vi "test.vi"(8 "Voie physique DAQmx 2":tag="sHIT/ai0") -> ()   [LabVIEW 2013]
uses:
  <vilib>/DAQmx/read.llb/DAQmx Read (Analog Wfm 1Chan NSamp).vi
  <vilib>/DAQmx/miscellaneous.llb/DAQmx Fill In Error Info.vi
  <vilib>/express/express analysis/Spectral/Block/exnSpectralBlock spectral measurements PSD poly.vi
  <vilib>/express/express analysis/Spectral/Block/exnSpectralBlock spectral measurements PSD WFM.vi
  <vilib>/express/express analysis/Spectral/XNode/ExpressSpectralMeasurementsBlockNode.xnode
panel:
  out "Final Waveform":waveform(dbl)(graph)
  in  "Fenetre d'affichage (s)":dbl step=0.001
  out "?":cluster{"f0":dbl, "df":dbl, "magnitude":dbl[]}(graph)
  in  "FFT":bool
  out "Frequence":dbl
  out "Valeur eff":dbl
  out "Moyenne":dbl
  in  "Statistiques":bool
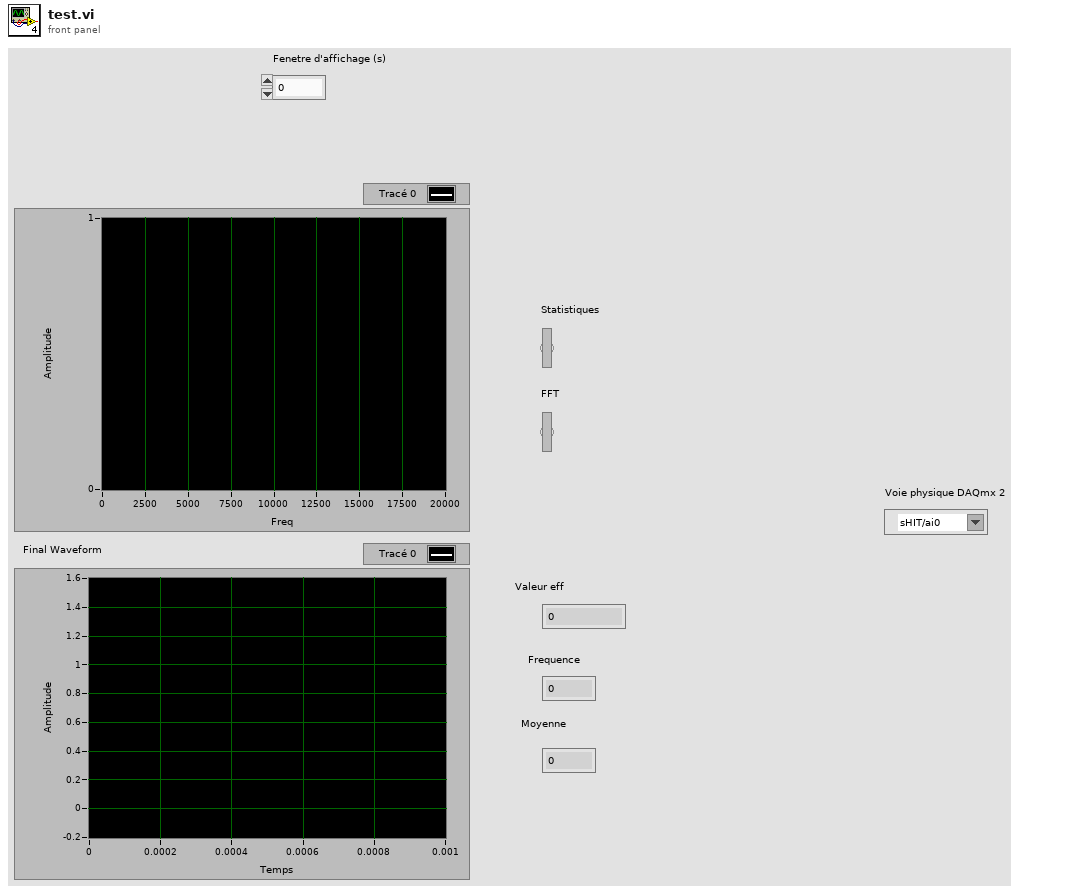
[diagram p1: front panel]
types:
  T1 = cluster{"averaging mode":u16, "weighting mode":u16, "number of averages":u32}
  T2 = cluster{"dB On (F)":bool, "unwrap phase (F)":bool, "convert to degree (F)":bool}
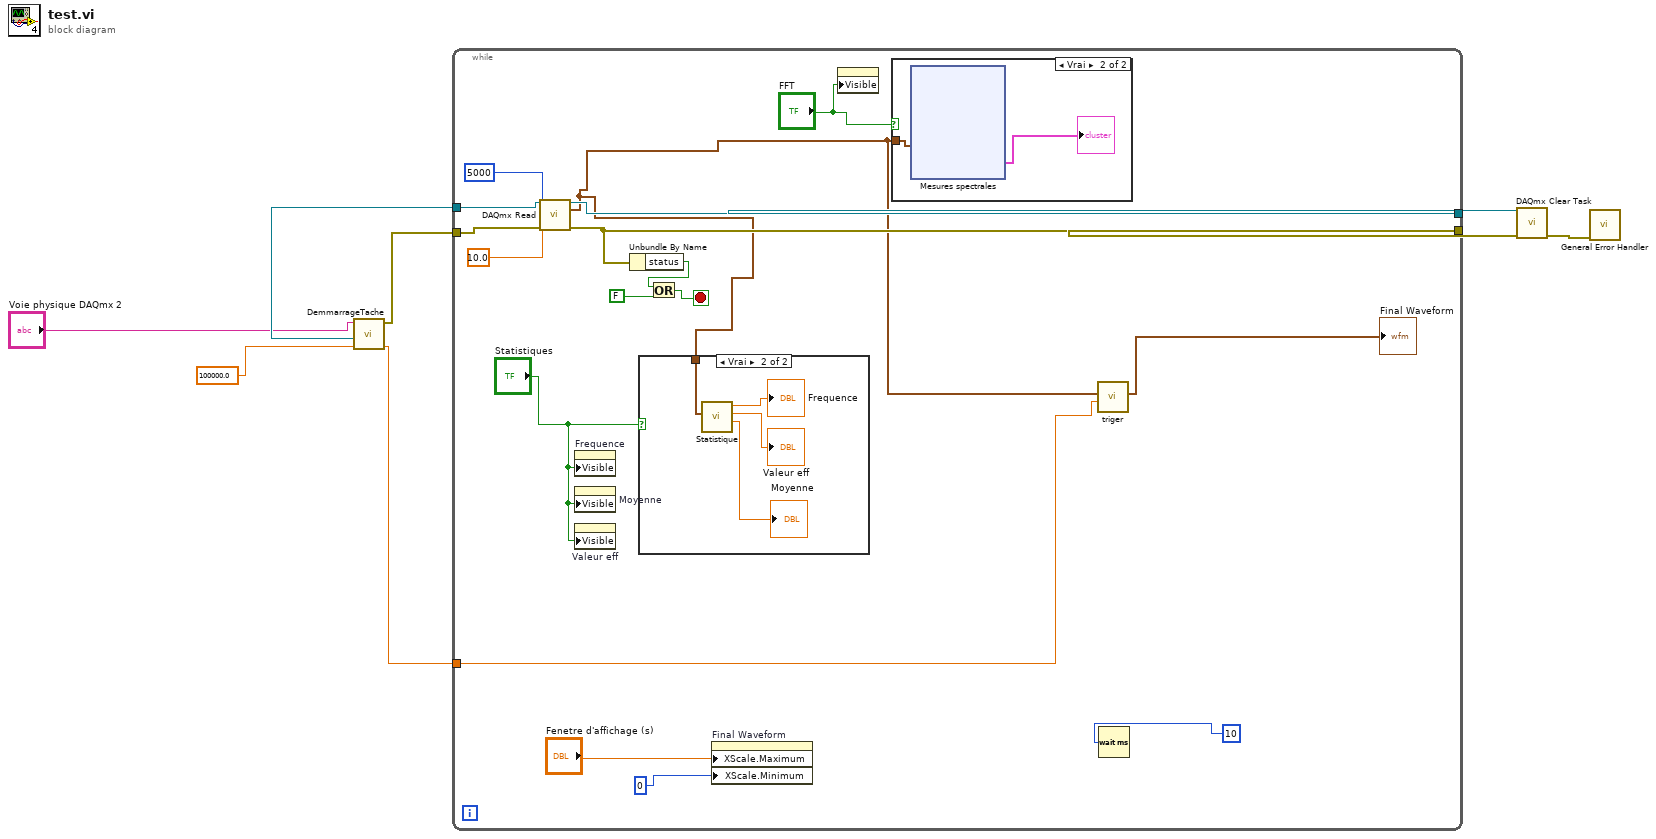
[diagram p0: block diagram]
diagram:
  n1 = call "DemmarrageTache.vi"("frequence echantillonage"=100000.0, "Voie physique DAQmx"="Voie physique DAQmx 2") -> ("frequence echantillonage 2"=w2:dbl, "task out"=w3:refnum<k21>, "error out"=w4:errorcluster)  [unwired: 6 in]
  n2 = while {
    tunnel: w3 -> [w25]
    tunnel: w4 -> [w24]
    tunnel: [w22] -> w8
    tunnel: [w18] -> w7
    tunnel: w2 -> [w9]
    stop <- w21 stop-if-true
    n3 = call-poly <vilib>:"DAQmx Read.vi"("task/channels in"=w25, "number of samples per channel"=5000, "timeout"=10.0, "error in"=w24) -> ("task out"=w22:refnum<k21>, "data"=w11:waveform(dbl), "error out"=w18:errorcluster)  [unwired: 9 in]
    n4 = property on="Frequence" class="NumNb (strict)"("Visible"="Statistiques") -> ()  [unwired: 2 in, 2 out]
    n5 = property on="Moyenne" class="NumNb (strict)"("Visible"="Statistiques") -> ()  [unwired: 2 in, 2 out]
    n6 = property on="Valeur eff" class="NumNb (strict)"("Visible"="Statistiques") -> ()  [unwired: 2 in, 2 out]
    n7 = Unbundle By Name(w18) -> ("status"=w19:bool)
    n8 = case shown="Vrai" "Statistiques" {
      tunnel: w11 -> [_ w29]
      frame False {
      }
      frame True {
        n9 = call "Statistique.vi"("Waveform"=w29) -> ("mean"=→"Moyenne":dbl, "Valeur efficace"=→"Valeur eff":dbl, "Fréquence"=→"Frequence":dbl)  [unwired: 8 in]
      }
    }
    n10 = Or(x=w19, y=FALSE) -> (x .or. y?=w21:bool)
    n11 = property on="Final Waveform" class="GraphWF (strict)"("XScale.Maximum"="Fenetre d'affichage (s)", "XScale.Minimum"=0) -> ()  [unwired: 2 in, 2 out]
    n12 = property class="GraphWF (strict)"("Visible"="FFT") -> ()  [unwired: 2 in, 2 out]
    n13 = case shown="Vrai" "FFT" {
      tunnel: w11 -> [_ w30]
      frame False {
      }
      frame True {
        n14 = xnode "Mesures spectrales"("Signaux"=w30) -> ("DSP"=→"?":cluster{"f0":dbl, "df":dbl, "magnitude":dbl[]})  [unwired: 1 in, 1 out]
      }
    }
    n15 = call "triger.vi"("frequene echantillonage"=w9, "Signal"=w11) -> ("waveform en sortie"=→"Final Waveform":waveform(dbl))  [unwired: 9 in]
    n16 = Wait (ms)(milliseconds to wait=10) -> ()  [unwired: 1 out]
  }
  n17 = call <vilib>:"DAQmx Clear Task.vi"("task in"=w8, "error in"=w7) -> ("error out"=w6:errorcluster)  [unwired: 13 in]
  n18 = call <vilib>:"General Error Handler.vi"("error in (no error)"=w6) -> ()  [unwired: 10 in, 5 out]
